vi "ProcedimentPrevi.vi"(6 "Quitar Pantalla":refnum<vi>, 8 "Pantalla retirada":refnum<vi>, 9 "Pantalla colocada":refnum<vi>, 10 "HORNO":refnum<vi>, 11 "Poner Pantalla":refnum<vi>) -> ()   [LabVIEW 2017]
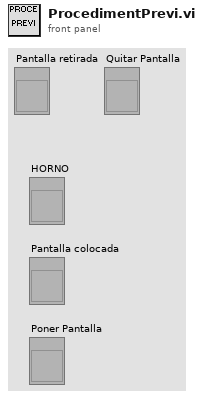
[diagram p1: front panel]
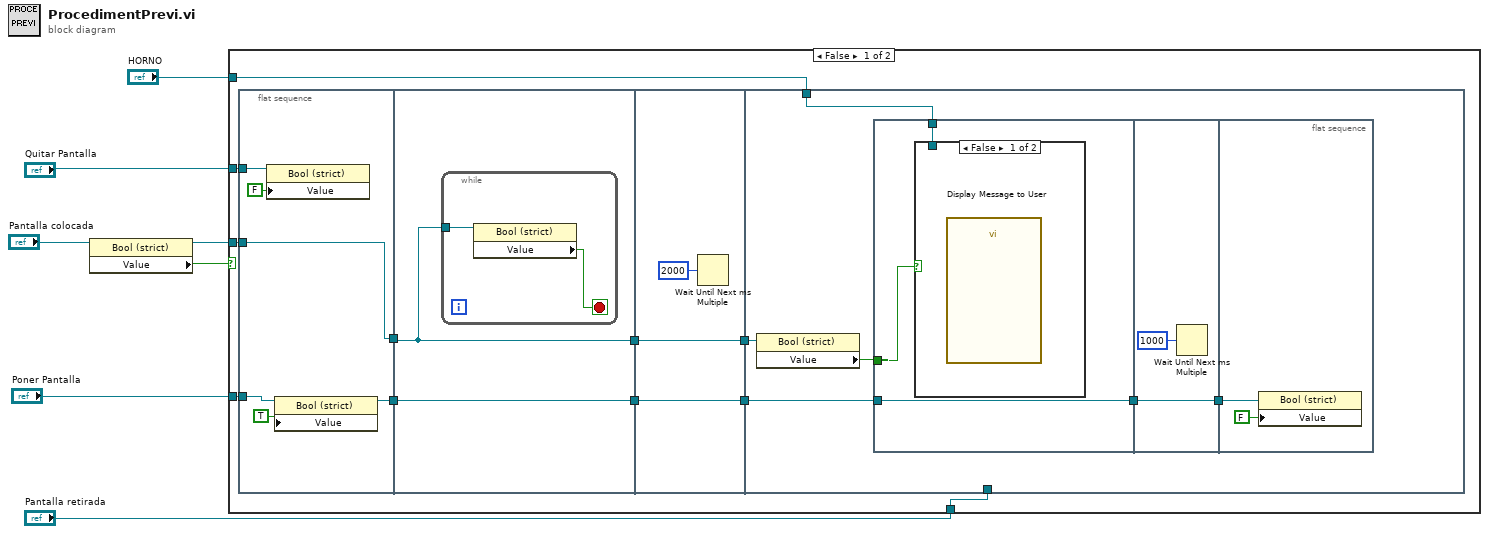
[diagram p0: block diagram]
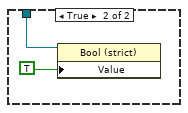
[diagram p2: hidden frame]
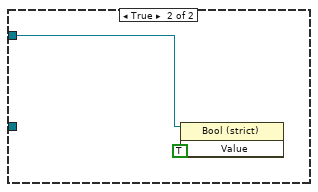
[diagram p3: hidden frame]
diagram:
  n1 = property class="Bool (strict)"(reference="Pantalla colocada") -> (reference out=w3:refnum<vi>, "Value"=w6:bool)  [unwired: 1 in, 1 out]
  n2 = case shown="False" w6 {
    tunnel: "HORNO" -> [w18 w47]
    tunnel: "Poner Pantalla" -> [w17 _]
    tunnel: w3 -> [w15 _]
    tunnel: "Pantalla retirada" -> [w13 _]
    tunnel: "Quitar Pantalla" -> [w12 _]
    frame False {
      n3 = flat-sequence {
        tunnel: w17 -> [w24]
        tunnel: [w22] -> w16
        tunnel: w15 -> [w22]
        tunnel: [w21] -> w14
        tunnel: w12 -> [w20]
        tunnel: w16 -> [w25]
        tunnel: [w26] -> w11
        tunnel: w14 -> [w26]
        tunnel: [w25] -> w9
        tunnel: w11 -> [w31]
        tunnel: [w31] -> w10
        tunnel: w9 -> [w30]
        tunnel: [w30] -> w8
        tunnel: w18 -> [w37]
        tunnel: w10 -> [w36]
        tunnel: w13 -> [_]
        tunnel: w8 -> [w35]
        frame #0 {
          n4 = property class="Bool (strict)"(reference=w20, "Value"=FALSE) -> ()  [unwired: 1 in, 2 out]
          n5 = property class="Bool (strict)"(reference=w24, "Value"=TRUE) -> (reference out=w21:refnum<vi>)  [unwired: 1 in, 1 out]
        }
        frame #1 {
          n6 = while {
            tunnel: w25 -> [w28]
            stop <- w27 stop-if-true
            n7 = property class="Bool (strict)"(reference=w28) -> ("Value"=w27:bool)  [unwired: 1 in, 2 out]
          }
        }
        frame #2 {
          n8 = Wait Until Next ms Multiple(millisecond multiple=u32 2000) -> ()  [unwired: 1 out]
        }
        frame #3 {
          n9 = property on="Property Node" class="Bool (strict)"(reference=w35) -> ("Value"=w34:bool)  [unwired: 1 in, 2 out]
          n10 = flat-sequence {
            tunnel: w37 -> [w40]
            tunnel: [w39] -> w33
            tunnel: w36 -> [w39]
            tunnel: w34 -> [w38]
            tunnel: w33 -> [w44]
            tunnel: [w44] -> w32
            tunnel: w32 -> [w45]
            frame #0 {
              n11 = case shown="False" w38 {
                tunnel: w40 -> [_ w41]
                frame False {
                  n12 = call "Display Message to User"() -> ()  [unwired: 10 in, 2 out]
                }
                frame True {
                  n13 = property class="Bool (strict)"(reference=w41, "Value"=TRUE ("HORNO")) -> ()  [unwired: 1 in, 2 out]
                }
              }
            }
            frame #1 {
              n14 = Wait Until Next ms Multiple(millisecond multiple=u32 1000) -> ()  [unwired: 1 out]
            }
            frame #2 {
              n15 = property class="Bool (strict)"(reference=w45, "Value"=FALSE) -> ()  [unwired: 1 in, 2 out]
            }
          }
        }
      }
    }
    frame True {
      n16 = property class="Bool (strict)"(reference=w47, "Value"=TRUE ("HORNO")) -> ()  [unwired: 1 in, 2 out]
    }
  }
